vi "VisionLab_ShoreFollow_Main.vi"() -> ()   [LabVIEW 2014]
uses:
  <vilib>/vision/Image Controls.llb/IMAQ Image.ctl
  <vilib>/userdefined/High Color/IMAQdx.ctl
  <vilib>/vision/driver/NI_Vision_Acquisition_Software.lvlib
panel:
  in  "Destination Point":cluster{"DestinationX":dbl, "DestinationY":dbl}={"DestinationX"=520.0, "DestinationY"=320.0}
  out "LH_Find":T1
  out "servo error out":errorcluster
  out "error out":errorcluster
  out "Live Input":T1(plugin-control)
  out "Running":bool
  in  "stop":bool
  out "FindLaser Out":T1(plugin-control)
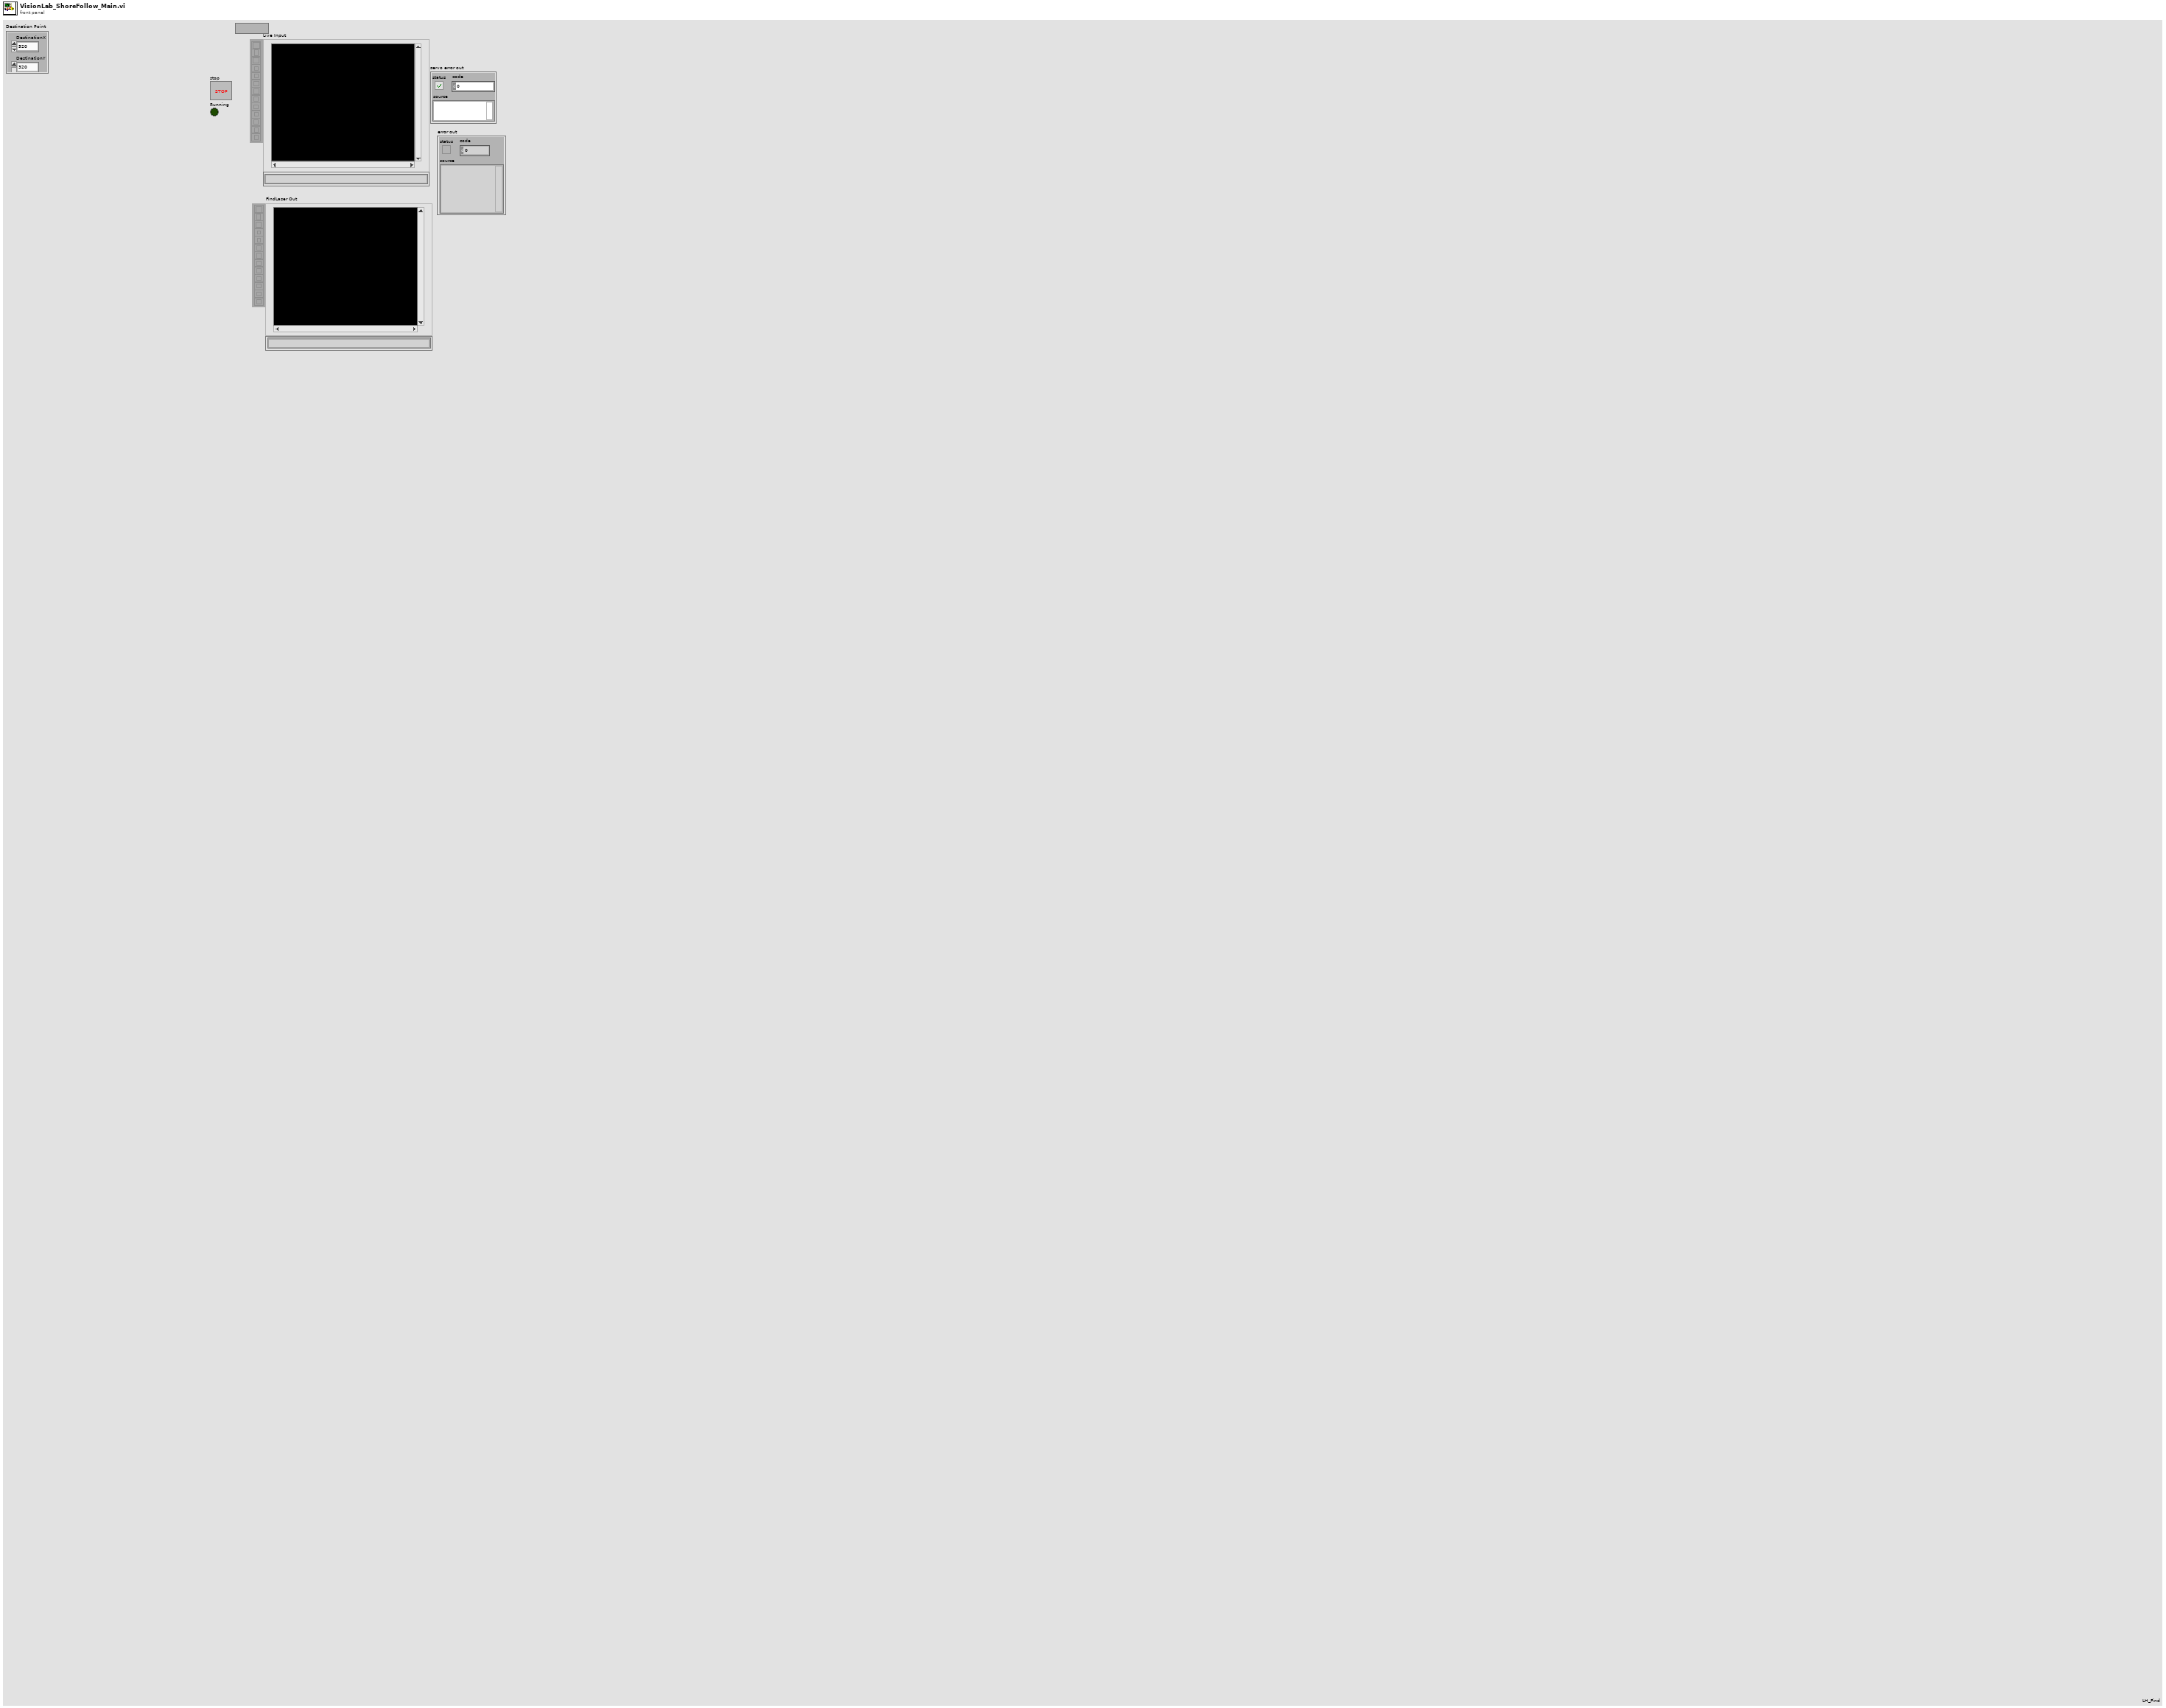
[diagram p1: front panel]
types:
  T1 = typedef "IMAQ Image.ctl" = refnum<image>
  T2 = typedef "IMAQdx.ctl" = refnum<k21>
  T3 = typedef "Image Type" = u32
  T4 = cluster{"Point1 (Pixels)":cluster{"X":sgl, "Y":sgl}, "Point2 (Pixels)":cluster{"X":sgl, "Y":sgl}, "Point1 (Real-World)":cluster{"X":sgl, "Y":sgl}, "Point2 (Real-World)":cluster{"X":sgl, "Y":sgl}, "Angle (Pixel)":dbl, "Angle (Real-World)":dbl, "Score":dbl, "Straightness":dbl, "Average SNR (db)":dbl, "Calibration Valid":bool}
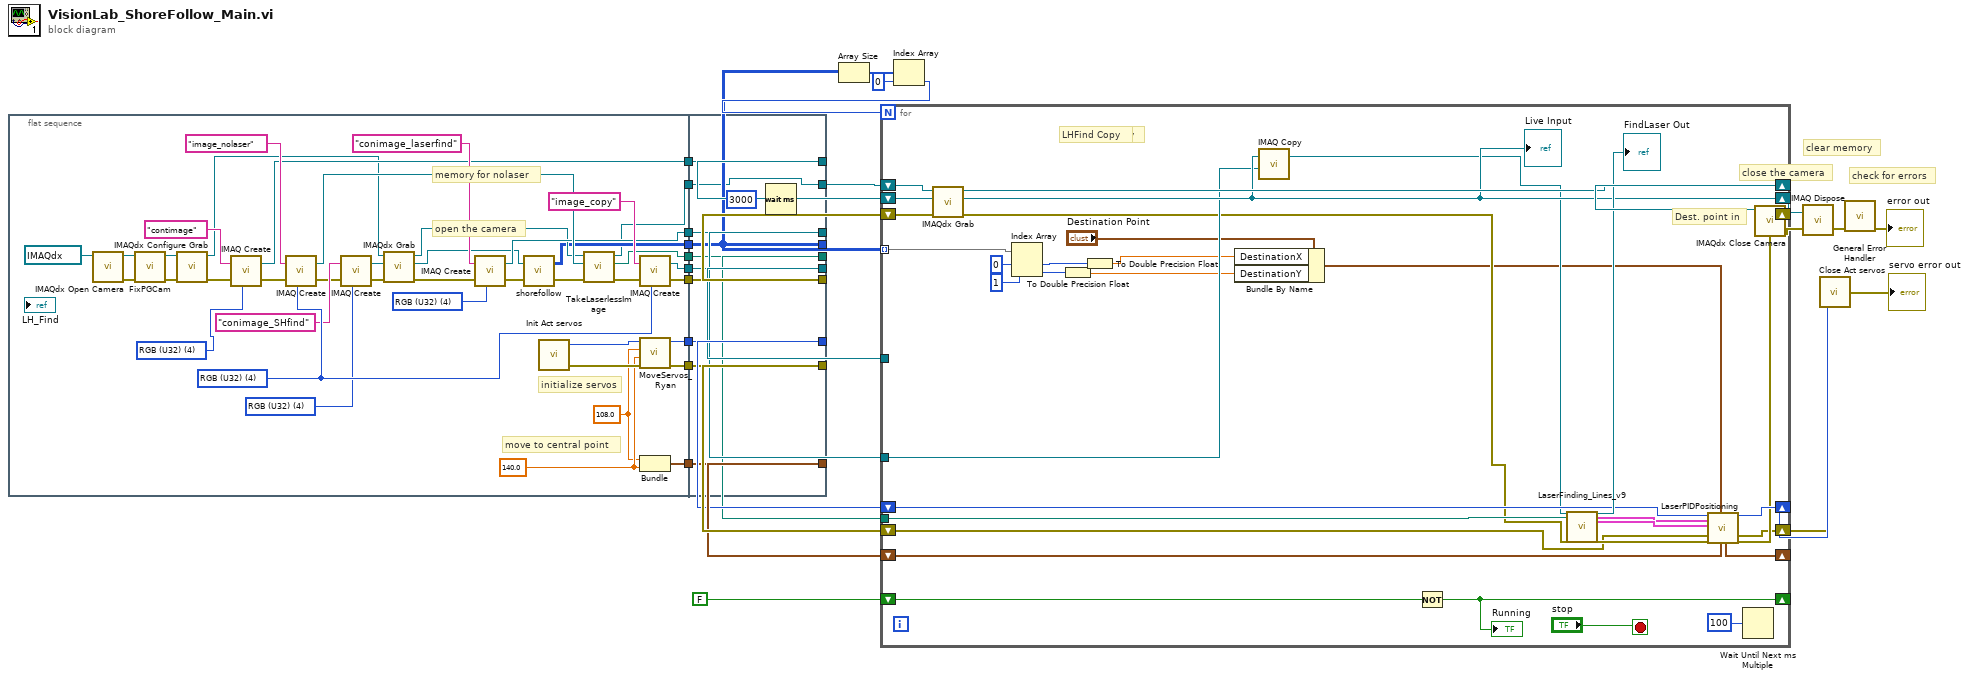
[diagram p0: block diagram]
diagram:
  # "check for errors"
  # "clear memory"
  # "close the camera"
  n1 = flat-sequence {
    tunnel: [w54] -> w11
    tunnel: [w45] -> w10
    tunnel: [w65] -> w9
    tunnel: [w63] -> w8
    tunnel: [w60] -> w7
    tunnel: [w53] -> w6
    tunnel: [w47] -> w5
    tunnel: [w46] -> w4
    tunnel: [w35] -> w3
    tunnel: [w34] -> w2
    tunnel: [w77] -> w12
    tunnel: [w78] -> w16
    tunnel: [w79] -> w17
    tunnel: [w80] -> w18
    tunnel: [w81] -> w20
    tunnel: [w82] -> w22
    tunnel: [w83] -> w19
    tunnel: [w84] -> w26
    tunnel: [w85] -> w33
    tunnel: w11 -> [w85]
    tunnel: w10 -> [w84]
    tunnel: w9 -> [w83]
    tunnel: w8 -> [w82]
    tunnel: w7 -> [w81]
    tunnel: w6 -> [w80]
    tunnel: w5 -> [w79]
    tunnel: w4 -> [w78]
    tunnel: w3 -> [w77]
    tunnel: w2 -> [w75]
    tunnel: [w75] -> w1
    frame #0 {
      w48 = T3 4 items=["Grayscale (U8)", "Grayscale (I16)", "Grayscale (SGL)", "Complex (CSG)", "RGB (U32)", "HSL (U32)", "RGB (U64)", "Grayscale (U16)"] ("Image Type")
      w51 = T3 4 items=["Grayscale (U8)", "Grayscale (I16)", "Grayscale (SGL)", "Complex (CSG)", "RGB (U32)", "HSL (U32)", "RGB (U64)", "Grayscale (U16)"] ("Image Type")
      w55 = T3 4 items=["Grayscale (U8)", "Grayscale (I16)", "Grayscale (SGL)", "Complex (CSG)", "RGB (U32)", "HSL (U32)", "RGB (U64)", "Grayscale (U16)"] ("Image Type")
      w61 = 108.0 ("Y pos")
      w62 = 140.0 ("X pos")
      w72 = T3 4 items=["Grayscale (U8)", "Grayscale (I16)", "Grayscale (SGL)", "Complex (CSG)", "RGB (U32)", "HSL (U32)", "RGB (U64)", "Grayscale (U16)"] ("Image Type")
      # "memory for nolaser"
      # "move to central point"
      # "initialize servos"
      # "open the camera"
      n2 = call <vilib>:"IMAQdx Open Camera.vi"("Session In"=T2 "cam1") -> ("error out"=w68:errorcluster, "Session Out"=w67:T2)  [unwired: 2 in, 7 out]
      n3 = call "FixPGCam.vi"("error in"=w68, "Session In"=w67) -> ("error out"=w70:errorcluster, "IMAQdx Session Out"=w69:T2)  [unwired: 8 in]
      n4 = call <vilib>:"IMAQdx Configure Grab.vi"("error in"=w70, "Session In"=w69) -> ("error out"=w71:errorcluster, "Session Out"=w41:T2)  [unwired: 8 out]
      n5 = call "IMAQ Create"("Image Name"="contimage", "Image Type"=w72, "error in (no error)"=w71) -> ("New Image"=w45:T1, "error out"=w59:errorcluster)  [unwired: 1 in, 1 out]
      n6 = call "IMAQ Create"("Image Name"="image_nolaser", "Image Type"=w55, "error in (no error)"=w59) -> ("New Image"=w57:T1, "error out"=w50:errorcluster)  [unwired: 1 in, 1 out]
      n7 = call "IMAQ Create"("Image Name"="conimage_SHfind", "Image Type"=w51, "error in (no error)"=w50) -> ("New Image"=w39:T1, "error out"=w43:errorcluster)  [unwired: 1 in, 1 out]
      n8 = call <vilib>:"IMAQdx Grab.vi"("error in"=w43, "Image In"=w39, "Session In"=w41) -> ("error out"=w42:errorcluster, "Image Out"=w38:T1, "Session Out"=w40:T2)  [unwired: 1 in, 5 out]
      n9 = call "IMAQ Create"("Image Name"="conimage_laserfind", "Image Type"=w48, "error in (no error)"=w42) -> ("New Image"=w47:T1, "error out"=w37:errorcluster)  [unwired: 1 in, 1 out]
      n10 = call "shorefollow.vi"("error in (no error)"=w37, "Image in"=w38) -> ("error out"=w36:errorcluster, "Ordered Coordinates"=w35:i32[][])
      n11 = call "Init Act servos.vi"() -> ("Device Out"=w66:i32, "error out"=w64:errorcluster)  [unwired: 1 in, 1 out]
      n12 = call "TakeLaserlessImage.vi"("error in"=w36, "Image In"=w57, "Session In"=w40) -> ("error out"=w44:errorcluster, "nolaser Filepath"=w46:path, "Session Out"=w34:T2)  [unwired: 6 in]
      n13 = call "IMAQ Create"("Image Name"="image_copy", "Image Type"=w55, "error in (no error)"=w44) -> ("New Image"=w53:T1, "error out"=w54:errorcluster)  [unwired: 2 in]
      n14 = call "MoveServos_Ryan.vi"("servo error in"=w64, "Y pos"=w62, "X pos"=w61, "Device In"=w66) -> ("servo error out"=w63:errorcluster, "Device Out"=w65:i32)  [unwired: 6 in]
      n15 = Bundle("Y pos"=w61, "X pos"=w62) -> (w60:cluster{"Y pos":dbl, "X pos":dbl})  [unwired: 1 in]
    }
    frame #1 {
      n16 = Wait (ms)(milliseconds to wait=u32 3000) -> ()  [unwired: 1 out]
    }
  }
  n17 = Array Size(array=w12) -> (size(s)=w15:i32[])
  n18 = Index Array(array=w15, index=0) -> (element=w13:i32)
  n19 = for {
    N: w13 -> [_]
    shift-right: [w115] -> w32
    shift-left: w1 -> [w117]
    shift-right: [w100] -> w30
    shift-left: w26 -> [w111]
    shift-right: [w105] -> w24
    shift-left: w33 -> [w116]
    shift-right: [w113] -> _
    shift-left: FALSE -> [w114]
    shift-right: [w108] -> w25
    shift-left: w19 -> [w101]
    shift-right: [w107] -> _
    shift-left: w20 -> [w106]
    shift-right: [w102] -> w21
    shift-left: w22 -> [w103]
    tunnel: w18 -> [_]
    tunnel: w17 -> [w99]
    tunnel: w16 -> [w97]
    tunnel: w12 -> [w95] mode=indexing
    stop <- "stop" stop-if-true
    # "LaserFind Copy"
    # "LHFind Copy"
    # "Dest. point in"
    n20 = call <vilib>:"IMAQdx Grab.vi"("error in"=w116, "Image In"=w111, "Session In"=w117) -> ("error out"=w96:errorcluster, "Image Out"=w100:T1, "Session Out"=w115:T2)  [unwired: 1 in, 5 out]
    "Live Input" <- w100
    n21 = Index Array(array=w95, index #1=0 ("index"), index #2=1 ("index")) -> (element #1=w92:i32, element #2=w91:i32)
    n22 = To Double Precision Float(number=w91) -> (double precision float=w88:dbl)
    n23 = To Double Precision Float(number=w92) -> (double precision float=w89:dbl)
    n24 = Bundle By Name(cluster="Destination Point", "DestinationX"=w89, "DestinationY"=w88) -> (w90:cluster{"DestinationX":dbl, "DestinationY":dbl})
    n25 = call "IMAQ Copy"("Image Dst"=w99, "Image Src"=w100) -> ("Image Dst Out"=w98:T1)  [unwired: 4 in, 1 out]
    n26 = Not(x=w114) -> (.not. x?=w113:bool)
    "Running" <- w113
    n27 = call "LaserFinding_Lines_v9.vi"("Image In"=w98, "File Path (Get Image without Laser)"=w97, "error in"=w96) -> ("Image Out"=→"FindLaser Out":T1, "Straight Edge (Find Vert. Edge)"=w109:T4, "Straight Edge (Find Horiz. Edge)"=w110:T4, "error out"=w104:errorcluster)  [unwired: 21 in]
    n28 = call "LaserPIDPositioning.vi"("Servo Device In"=w101, "Vertical Edge"=w109, "Horizontal Edge"=w110, "servo error in"=w103, "error in"=w104, "Destination Point"=w90, "Servo Angles In"=w106) -> ("Servo Angles Out"=w107:cluster{"Angle X":dbl, "Angle Y":dbl}, "Servo Device Out"=w108:i32, "servo error out"=w102:errorcluster, "error out"=w105:errorcluster)  [unwired: 9 in]
    n29 = Wait Until Next ms Multiple(millisecond multiple=u32 100 ("milliseconds to wait")) -> ()  [unwired: 1 out]
  }
  n30 = call <vilib>:"IMAQdx Close Camera.vi"("error in"=w24, "Session In"=w32) -> ("error out"=w31:errorcluster)  [unwired: 9 out]
  n31 = call "IMAQ Dispose"("Image"=w30, "error in (no error)"=w31) -> ("error out"=w29:errorcluster)  [unwired: 1 in, 3 out]
  n32 = call "Close Act servos.vi"("error in"=w21, "Device In"=w25) -> ("error out"=→"servo error out":errorcluster)
  n33 = call <vilib>:"General Error Handler.vi"("error in (no error)"=w29) -> ("error out"=→"error out":errorcluster)  [unwired: 2 in, 12 out]
